vi "SPI Sensor Processing.vi"(11 "stop":bool) -> ()   [LabVIEW 2014]
uses:
  <vilib>/rvi/interface/nirviOpenFPGA/nirviOpenFPGA.xnode
  FPGA/Sensor Library/FPGA.vi
  SPI/Controls/FPGA Reference.ctl
  Global Data.vi
  <vilib>/rvi/interface/nirviCloseFPGA/nirviCloseFPGA.xnode
  FPGA Bitfiles/FormulaElectric2_FPGATarget_FPGA_KFopRbsiCjk.lvbitx
  <vilib>/FPGAPlugInAG/sbRIO-9626/niLvFpga_Close_sbRIO-9626.vi
  FPGA Telemetry.ctl
  FPGA/SPI/Controls/FPGA SPI_FPGA SPI State.ctl
  <vilib>/FPGAPlugInAG/sbRIO-9626/niLvFpga_Open_sbRIO-9626.vi
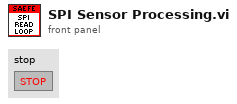
[diagram p1: front panel]
types:
  T1 = typedef "FPGA Reference.ctl" = refnum<k20>
  T2 = typedef "FPGA Telemetry.ctl" = cluster{"SPI":cluster{"SPI_Ack Read":bool, "SPI_Read Flag":bool, "SPI_Read Data":u8, "SPI_Write Data":u8, "SPI_Write Flag":bool, "SPI_Total Bytes":u16, "SPI_Total Bits":u16, "SPI_CS":u8, "SPI_CS Active State":bool, "SPI_Clock Divider":u32, "SPI_CPHA":bool, "SPI_CPOL":bool, "SPI_Cmd":T3, "SPI_Port":i8, "SPI_Start":bool, "Ready":bool}, "sbRIO":cluster{"Supply Voltage (V)":fxp<+/-,25,6>, "FPGA LED":bool, "Chassis Temperature":i16}, "Throttles":cluster{"Throttles Consistent?":bool, "Throttles In Range?":bool, "Average Throttle (%)":fxp<+/-,29,18>, "Throttle 2 (V)":fxp<+/-,24,5>, "Throttle 2 (%)":fxp<+/-,27,18>, "Throttle 1 (V)":fxp<+/-,24,5>, "Throttle 1 (%)":fxp<+/-,27,18>, "Throttle 2 Max":fxp<+,16,4>, "Throttle 2 Min":fxp<+,16,4>, "Throttle 1 Max":fxp<+,16,4>, "Throttle 1 Min":fxp<+,16,4>}, "Loads & Shutdown":cluster{"RTDS Enable":bool, "TSMS Status":bool, "Positive AIR Enable":bool, "cRIO Shutdown 2":bool, "cRIO Shutdown 1":bool, "Latch Status":bool, "Coolant Pump":bool, "Red Dash LED":bool, "Yellow Dash LED":bool, "Green Dash LED":bool, "BMS OK":bool, "IMD In":bool, "BSPD In":bool, "Brake Light Out":bool}, "Motor Controller":cluster{"Motor Controller Dash Switch":bool, "Motor Controller Enable":bool}, "Sensors":cluster{"RL Tick Period":u32, "RR Tick Period":u32, "FR Tick Period":u32, "FL Tick Period":u32, "RR Shock (V)":fxp<+/-,24,5>, "RL Shock (V)":fxp<+/-,24,5>, "FR Shock (V)":fxp<+/-,24,5>, "FL Shock (V)":fxp<+/-,24,5>, "RR Stopped":bool, "RL Stopped":bool, "FR Stopped":bool, "FL Stopped":bool, "Steering Wheel Middle":fxp<+/-,26,5>, "Steering Wheel Angle (degrees)":fxp<+/-,31,13>, "High Current OK?":bool, "Low Current OK?":bool, "Rear BPS OK?":bool, "Front BPS OK?":bool, "Rear BP (psi)":fxp<+/-,27,16>, "Front BP (psi)":fxp<+/-,27,16>, "High Current (A)":fxp<+/-,24,15>, "Low Current (A)":fxp<+/-,24,15>}}
  T3 = typedef "FPGA SPI_FPGA SPI State.ctl" = enum8{"Idle", "Read/Write SPI", "Configure"}
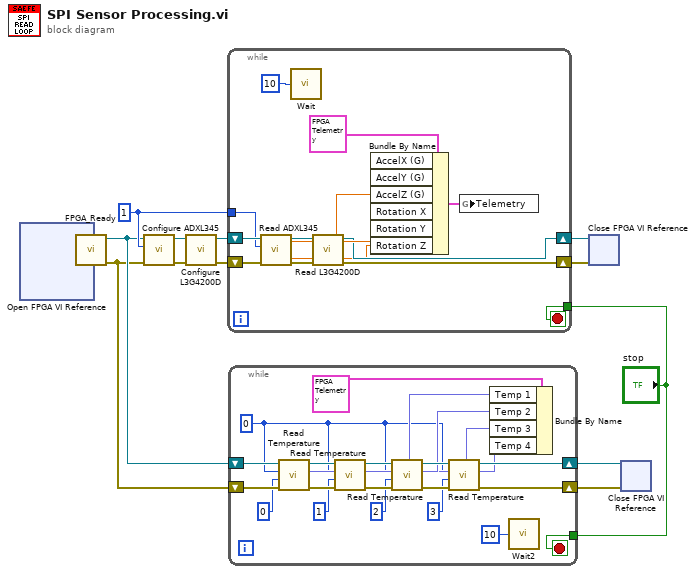
[diagram p0: block diagram]
diagram:
  w12 = i8 1 ("Port")
  n1 = xnode "Open FPGA VI Reference"() -> ("FPGA VI Reference Out"=w14:T1, "error out"=w13:errorcluster)  [unwired: 2 in]
  n2 = call "FPGA_Ready.vi"("Error In"=w13, "FPGA VI Reference In"=w14) -> ("Error Out"=w4:errorcluster, "FPGA VI Reference Out"=w5:T1)  [unwired: 7 in]
  n3 = call "Configure ADXL345.vi"("error in"=w4, "Port"=w12, "FPGA VI Reference"=w5) -> ("error out"=w8:errorcluster, "FPGA VI Reference Out"=w9:T1)  [unwired: 7 in]
  n4 = call "Configure L3G4200D.vi"("error in"=w8, "FPGA VI Reference"=w9) -> ("error out"=w10:errorcluster, "FPGA VI Reference Out"=w11:T1)  [unwired: 8 in]
  n5 = while {
    tunnel: w12 -> [w29]
    shift-right: [w22] -> w6
    shift-left: w10 -> [w30]
    shift-right: [w23] -> w7
    shift-left: w11 -> [w31]
    tunnel: "stop" -> [w15]
    stop <- w15 stop-if-true
    n6 = call "Read ADXL345.vi"("Error In"=w30, "Port"=w29, "FPGA VI Reference In"=w31) -> ("error out"=w24:errorcluster, "FPGA VI Reference Out"=w25:T1, "Y"=w27:dbl, "Z"=w26:dbl, "X"=w28:dbl)  [unwired: 4 in]
    n7 = call "Wait"("Count(mSec)"=u32 10) -> ()  [unwired: 1 out]
    n8 = call "Read L3G4200D.vi"("Error In"=w24, "FPGA VI Reference In"=w25) -> ("error out"=w22:errorcluster, "FPGA VI Reference Out"=w23:T1, "Z Rotation Rate (mdps)"=w19:dbl, "Y Rotation Rate (mdps)"=w20:dbl, "X Rotation Rate (mdps)"=w21:dbl)  [unwired: 5 in]
    n9 = Bundle By Name(cluster=T2 {"SPI"={"SPI_Ack Read"=FALSE, "SPI_Read Flag"=FALSE, "SPI_Read Data"=0, "SPI_Write Data"=0, "SPI_Write Flag"=FALSE, "SPI_Total Bytes"=1, "SPI_Total Bits"=0, "SPI_CS"=0, "SPI_CS Active State"=FALSE, "SPI_Clock Divider"=0, "SPI_CPHA"=FALSE, "SPI_CPOL"=FALSE, "SPI_Cmd"=enum."Configure", "SPI_Port"=0, "SPI_Start"=FALSE, "Ready"=FALSE}, "sbRIO"={"Supply Voltage (V)"=0.0, "FPGA LED"=FALSE, "Chassis Temperature"=0}, "Throttles"={"Throttles Consistent?"=FALSE, "Throttles In Range?"=FALSE, "Average Throttle (%)"=185.44775390625, "Throttle 2 (V)"=0.0, "Throttle 2 (%)"=-866.732421875, "Throttle 1 (V)"=15.999998092651367, "Throttle 1 (%)"=0.34765625, "Throttle 2 Max"=0.0, "Throttle 2 Min"=0.0, "Throttle 1 Max"=0.0, "Throttle 1 Min"=0.0}, "Loads & Shutdown"={"RTDS Enable"=FALSE, "TSMS Status"=FALSE, "Positive AIR Enable"=FALSE, "cRIO Shutdown 2"=TRUE, "cRIO Shutdown 1"=TRUE, "Latch Status"=FALSE, "Coolant Pump"=FALSE, "Red Dash LED"=FALSE, "Yellow Dash LED"=FALSE, "Green Dash LED"=FALSE, "BMS OK"=FALSE, "IMD In"=FALSE, "BSPD In"=FALSE, "Brake Light Out"=TRUE}, "Motor Controller"={"Motor Controller Dash Switch"=TRUE, "Motor Controller Enable"=TRUE}, "Sensors"={"RL Tick Period"=0, "RR Tick Period"=0, "FR Tick Period"=0, "FL Tick Period"=0, "RR Shock (V)"=0.0, "RL Shock (V)"=0.0, "FR Shock (V)"=0.0, "FL Shock (V)"=0.0, "RR Stopped"=TRUE, "RL Stopped"=TRUE, "FR Stopped"=TRUE, "FL Stopped"=TRUE, "Steering Wheel Middle"=0.0, "Steering Wheel Angle (degrees)"=0.0, "High Current OK?"=FALSE, "Low Current OK?"=FALSE, "Rear BPS OK?"=TRUE, "Front BPS OK?"=TRUE, "Rear BP (psi)"=0.0, "Front BP (psi)"=0.0, "High Current (A)"=0.0, "Low Current (A)"=0.0}} ("Telemetry"), "AccelX (G)"=w28, "AccelY (G)"=w27, "AccelZ (G)"=w26, "Rotation X"=w21, "Rotation Y"=w20, "Rotation Z"=w19) -> (w16:T2)
    n10 = global write "Global Data.vi" "Telemetry"(w16) -> ()
  }
  n11 = while {
    shift-right: [w42] -> w3
    shift-left: w5 -> [w53]
    shift-right: [w43] -> w2
    shift-left: w4 -> [w52]
    tunnel: "stop" -> [w51]
    stop <- w51 stop-if-true
    w36 = i8 0 ("Port")
    n12 = call "Read Temperature.vi"("Error In"=w52, "Thermocouple #"=u8 0, "Port"=w36, "FPGA VI Reference In"=w53) -> ("error out"=w46:errorcluster, "Temperature Out (C)"=w40:fxp<+,12,10>, "FPGA VI Reference Out"=w49:T1)  [unwired: 5 in]
    n13 = call "Read Temperature.vi"("Error In"=w46, "Thermocouple #"=u8 1, "Port"=w36, "FPGA VI Reference In"=w49) -> ("error out"=w45:errorcluster, "Temperature Out (C)"=w39:fxp<+,12,10>, "FPGA VI Reference Out"=w48:T1)  [unwired: 5 in]
    n14 = call "Read Temperature.vi"("Error In"=w45, "Thermocouple #"=u8 2, "Port"=w36, "FPGA VI Reference In"=w48) -> ("error out"=w44:errorcluster, "Temperature Out (C)"=w38:fxp<+,12,10>, "FPGA VI Reference Out"=w47:T1)  [unwired: 5 in]
    n15 = call "Read Temperature.vi"("Error In"=w44, "Thermocouple #"=u8 3, "Port"=w36, "FPGA VI Reference In"=w47) -> ("error out"=w43:errorcluster, "Temperature Out (C)"=w37:fxp<+,12,10>, "FPGA VI Reference Out"=w42:T1)  [unwired: 5 in]
    n16 = Bundle By Name(cluster=T2 {"SPI"={"SPI_Ack Read"=FALSE, "SPI_Read Flag"=FALSE, "SPI_Read Data"=0, "SPI_Write Data"=0, "SPI_Write Flag"=FALSE, "SPI_Total Bytes"=1, "SPI_Total Bits"=0, "SPI_CS"=0, "SPI_CS Active State"=FALSE, "SPI_Clock Divider"=0, "SPI_CPHA"=FALSE, "SPI_CPOL"=FALSE, "SPI_Cmd"=enum."Configure", "SPI_Port"=0, "SPI_Start"=FALSE, "Ready"=FALSE}, "sbRIO"={"Supply Voltage (V)"=0.0, "FPGA LED"=FALSE, "Chassis Temperature"=0}, "Throttles"={"Throttles Consistent?"=FALSE, "Throttles In Range?"=FALSE, "Average Throttle (%)"=185.44775390625, "Throttle 2 (V)"=0.0, "Throttle 2 (%)"=-866.732421875, "Throttle 1 (V)"=15.999998092651367, "Throttle 1 (%)"=0.34765625, "Throttle 2 Max"=0.0, "Throttle 2 Min"=0.0, "Throttle 1 Max"=0.0, "Throttle 1 Min"=0.0}, "Loads & Shutdown"={"RTDS Enable"=FALSE, "TSMS Status"=FALSE, "Positive AIR Enable"=FALSE, "cRIO Shutdown 2"=TRUE, "cRIO Shutdown 1"=TRUE, "Latch Status"=FALSE, "Coolant Pump"=FALSE, "Red Dash LED"=FALSE, "Yellow Dash LED"=FALSE, "Green Dash LED"=FALSE, "BMS OK"=FALSE, "IMD In"=FALSE, "BSPD In"=FALSE, "Brake Light Out"=TRUE}, "Motor Controller"={"Motor Controller Dash Switch"=TRUE, "Motor Controller Enable"=TRUE}, "Sensors"={"RL Tick Period"=0, "RR Tick Period"=0, "FR Tick Period"=0, "FL Tick Period"=0, "RR Shock (V)"=0.0, "RL Shock (V)"=0.0, "FR Shock (V)"=0.0, "FL Shock (V)"=0.0, "RR Stopped"=TRUE, "RL Stopped"=TRUE, "FR Stopped"=TRUE, "FL Stopped"=TRUE, "Steering Wheel Middle"=0.0, "Steering Wheel Angle (degrees)"=0.0, "High Current OK?"=FALSE, "Low Current OK?"=FALSE, "Rear BPS OK?"=TRUE, "Front BPS OK?"=TRUE, "Rear BP (psi)"=0.0, "Front BP (psi)"=0.0, "High Current (A)"=0.0, "Low Current (A)"=0.0}} ("Telemetry"), "Temp 1"=w40, "Temp 2"=w39, "Temp 3"=w38, "Temp 4"=w37) -> ()  [unwired: 1 out]
    n17 = call "Wait2"("Count(mSec)"=u32 10) -> ()  [unwired: 1 out]
  }
  n18 = xnode "Close FPGA VI Reference"("FPGA VI Reference In"=w7, "error in"=w6) -> ()  [unwired: 1 out]
  n19 = xnode "Close FPGA VI Reference"("FPGA VI Reference In"=w3, "error in"=w2) -> ()  [unwired: 1 out]
